vi "PLC.WriteValues.vi"(7 "Idx":i32, 8 "error in":errorcluster, 10 "Slot":i32, 11 "Data_in":T1={"Status"={"Idx"=0, "ConnRef"=0, "State"=enum."Off", "LiveBitTimer"=timestamp(0 s since 1904-01-01)}, "Sets"={"Enable"=FALSE, "IP"="", "Rack"=0, "Slot"=0, "LifeBitTimer_s"=0.0, "DataBlockAddr_PCStatus"=0, "DataBlockAddr_PLCStatus"=1, "DataBlockAddr_PLCNewData"=[], "DataBlockSize_PLCNewData"=[], "DataBlockAddr_PLCChangeOver"=[], "DataBlockSize_PLCChangeOver"=[], "DataBlockAddr_PCChangeOver"=[], "DataBlockAddr_PLCCheckStatus"=[], "DataBlockSize_PLCCheckStatus"=[], "DataBlockAddr_PCCheckStatus"=[], "System"=""}, "PCstatus"={"General"={"LifeBit"=FALSE, "DbRun"=FALSE}, "Stations"=[]}, "PLCstatus"={"General"={"LifeBit"=FALSE}, "Stations"=[]}}) -> (0 "error out":errorcluster, 3 "Data_out":T1={"Status"={"Idx"=0, "ConnRef"=0, "State"=enum."Off", "LiveBitTimer"=timestamp(0 s since 1904-01-01)}, "Sets"={"Enable"=FALSE, "IP"="", "Rack"=0, "Slot"=0, "LifeBitTimer_s"=0.0, "DataBlockAddr_PCStatus"=0, "DataBlockAddr_PLCStatus"=1, "DataBlockAddr_PLCNewData"=[], "DataBlockSize_PLCNewData"=[], "DataBlockAddr_PLCChangeOver"=[], "DataBlockSize_PLCChangeOver"=[], "DataBlockAddr_PCChangeOver"=[], "DataBlockAddr_PLCCheckStatus"=[], "DataBlockSize_PLCCheckStatus"=[], "DataBlockAddr_PCCheckStatus"=[], "System"=""}, "PCstatus"={"General"={"LifeBit"=FALSE, "DbRun"=FALSE}, "Stations"=[]}, "PLCstatus"={"General"={"LifeBit"=FALSE}, "Stations"=[]}})   [LabVIEW 2016]
doc: "Get test results (measurement values) from PLC and save to database\n\nWabco 2017 All right reserved\nAuthor: maciej.szupienko@wabco-auto.com"
uses:
  PLC.Data.ctl
  PLC.Data.Status.ctl
  PLC.State.ctl
  PLC.Data.Sets.ctl
  LowLevel/PLC.DataBlock.PCstatus.ctl
  LowLevel/PLC.DataBlock.PCstatus.General.ctl
  LowLevel/PLC.DataBlock.PCstatus.Station.ctl
  LowLevel/PLC.DataBlock.PLCstatus.ctl
  LowLevel/PLC.DataBlock.PLCstatus.General.ctl
  LowLevel/PLC.DataBlock.PLCstatus.Station.ctl
  LowLevel/PLC.DataBlock.PLCvalues.ctl
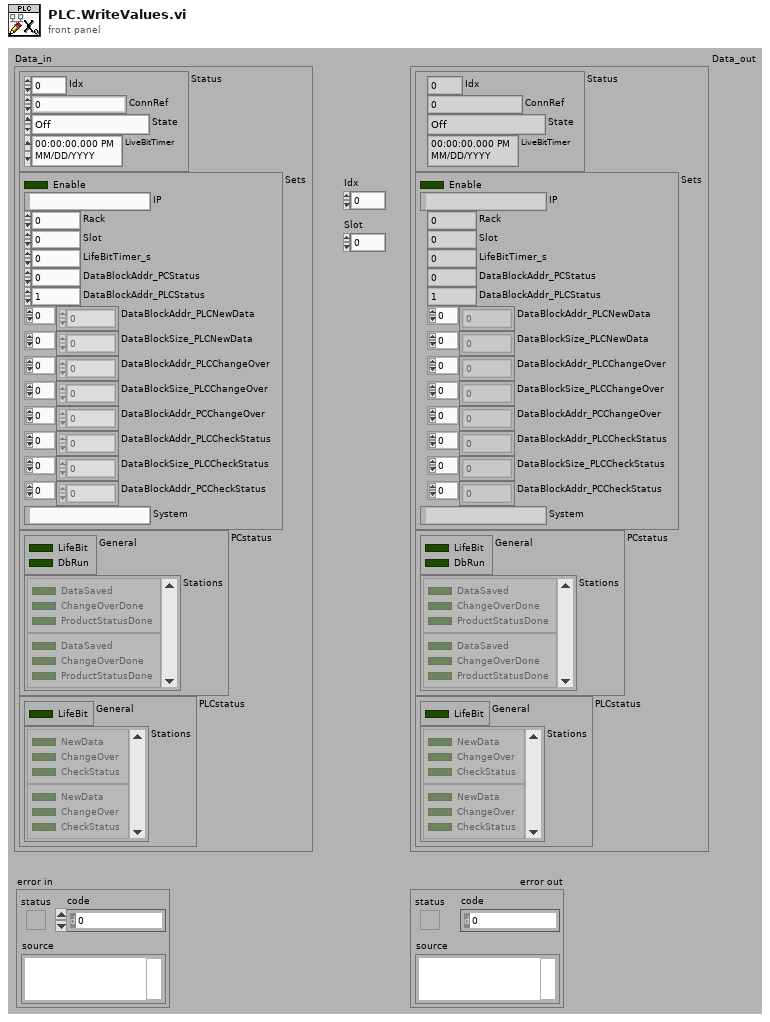
[diagram p1: front panel]
types:
  T1 = typedef "PLC.Data.ctl" = cluster{"Status":T2, "Sets":T4, "PCstatus":T5, "PLCstatus":T8}
  T2 = typedef "PLC.Data.Status.ctl" = cluster{"Idx":i32, "ConnRef":u64, "State":T3, "LiveBitTimer":timestamp}
  T3 = typedef "PLC.State.ctl" = enum32{"Off", "Error", "Idle", "Run"}
  T4 = typedef "PLC.Data.Sets.ctl" = cluster{"Enable":bool, "IP":string, "Rack":i32, "Slot":i32, "LifeBitTimer_s":dbl, "DataBlockAddr_PCStatus":i32, "DataBlockAddr_PLCStatus":i32, "DataBlockAddr_PLCNewData":i32[], "DataBlockSize_PLCNewData":i32[], "DataBlockAddr_PLCChangeOver":i32[], "DataBlockSize_PLCChangeOver":i32[], "DataBlockAddr_PCChangeOver":i32[], "DataBlockAddr_PLCCheckStatus":i32[], "DataBlockSize_PLCCheckStatus":i32[], "DataBlockAddr_PCCheckStatus":i32[], "System":string}
  T5 = typedef "PLC.DataBlock.PCstatus.ctl" = cluster{"General":T6, "Stations":T7[]}
  T6 = typedef "PLC.DataBlock.PCstatus.General.ctl" = cluster{"LifeBit":bool, "DbRun":bool}
  T7 = typedef "PLC.DataBlock.PCstatus.Station.ctl" = cluster{"DataSaved":bool, "ChangeOverDone":bool, "ProductStatusDone":bool}
  T8 = typedef "PLC.DataBlock.PLCstatus.ctl" = cluster{"General":T9, "Stations":T10[]}
  T9 = typedef "PLC.DataBlock.PLCstatus.General.ctl" = cluster{"LifeBit":bool}
  T10 = typedef "PLC.DataBlock.PLCstatus.Station.ctl" = cluster{"NewData":bool, "ChangeOver":bool, "CheckStatus":bool}
  T11 = typedef "PLC.DataBlock.PLCvalues.ctl" = cluster{"Status":u8, "Ref1":string, "Serial1":string, "Ref2":string, "Serial2":string, "Values":sgl[]}
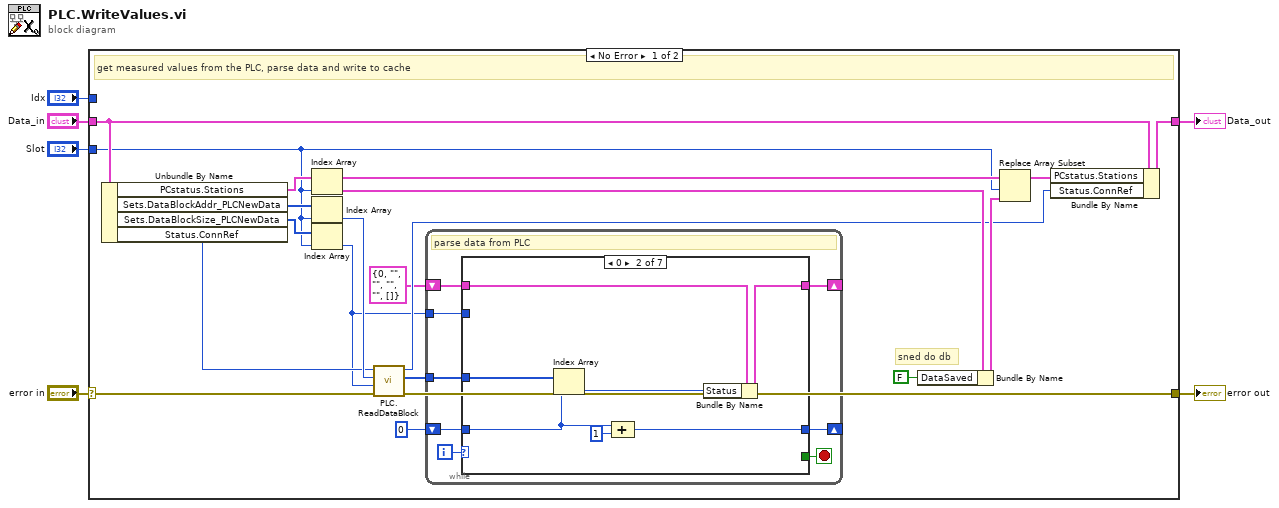
[diagram p0: block diagram]
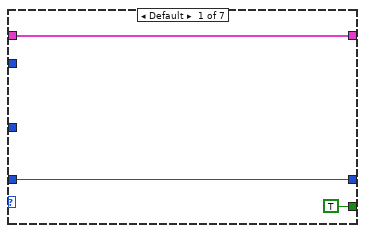
[diagram p2: hidden frame]
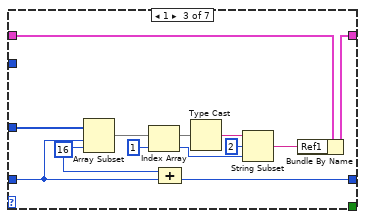
[diagram p3: hidden frame]
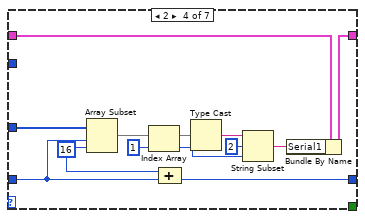
[diagram p4: hidden frame]
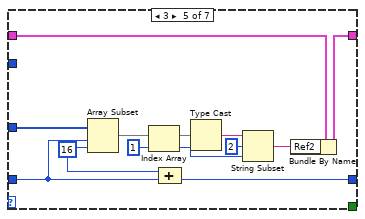
[diagram p5: hidden frame]
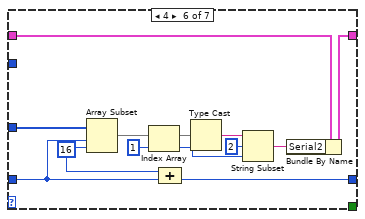
[diagram p6: hidden frame]
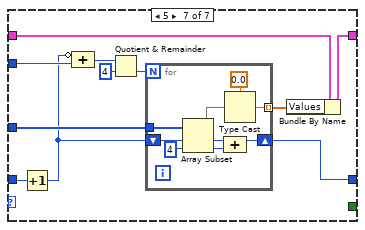
[diagram p7: hidden frame]
diagram:
  n1 = case shown="No Error" "error in" {
    selector: "error in" -> [w24 w111]
    tunnel: [w7 w111] -> w3
    tunnel: "Data_in" -> [w21 w110]
    tunnel: [w25 w110] -> w5
    tunnel: "Idx" -> [_ _]
    tunnel: "Slot" -> [w9 _]
    frame No Error {
      # "sned do db"
      # "get measured values from the PLC, parse data and write to cache"
      n2 = Unbundle By Name(w21) -> ("PCstatus.Stations"=w11:T7[], "Sets.DataBlockAddr_PLCNewData"=w23:i32[], "Sets.DataBlockSize_PLCNewData"=w10:i32[], "Status.ConnRef"=w20:u64)
      n3 = Index Array(array=w11, index=w9) -> (element=w18:T7)
      n4 = Index Array(array=w23, index=w9) -> (element=w22:i32)
      n5 = Index Array(array=w10, index=w9) -> (element=w12:i32)
      n6 = call "PLC.ReadDataBlock.vi"("error in (no error)"=w24, "Amount (1)"=w12, "Block"=w22, "Ref"=w20) -> ("error out"=w7:errorcluster, "data out"=w15:u8[], "ref out"=w16:u64)  [unwired: 5 in]
      n7 = while {
        tunnel: w15 -> [w28]
        shift-right: [w31] -> _
        shift-left: 0 -> [w32]
        shift-right: [w30] -> _
        shift-left: T11 {"Status"=0, "Ref1"="", "Serial1"="", "Ref2"="", "Serial2"="", "Values"=[]} ("element") -> [w29]
        tunnel: w12 -> [w27]
        i -> [w33]
        stop <- w26 stop-if-true
        # "parse data from PLC"
        n8 = case shown="0" w33 {
          tunnel: w32 -> [w35 w40 w46 w58 w70 w82 w93]
          tunnel: [w35 w41 w45 w57 w69 w81 w96] -> w31
          tunnel: [w36 w39 w55 w67 w79 w91 w101] -> w30
          tunnel: w29 -> [w36 w38 w54 w66 w78 w90 w102]
          tunnel: w28 -> [_ w43 w49 w61 w73 w85 w97]
          tunnel: w27 -> [_ _ _ _ _ _ w95]
          tunnel: [TRUE _ _ _ _ _ _] -> w26
          frame Default {
          }
          frame 0 {
            n9 = Index Array(array=w43, index=w40) -> (element=w42:u8)
            n10 = Compound Arithmetic op=ADD(w40, 1 ("value")) -> (w41:i32)
            n11 = Bundle By Name(cluster=w38, "Status"=w42) -> (w39:T11)
          }
          frame 1 {
            w47 = 16 ("length")
            n12 = Array Subset(array=w49, index=w46, length=w47) -> (w51:u8[])
            n13 = Index Array(array=w51, index=1) -> (element=w44:u8)
            n14 = Compound Arithmetic op=ADD(w47, w46) -> (w45:i32)
            n15 = Type Cast(x=w51) -> (*(type *) &x=w50:string)  [unwired: 1 in]
            n16 = String Subset(string=w50, offset (0)=2, length (rest)=w44) -> (substring=w48:string)
            n17 = Bundle By Name(cluster=w54, "Ref1"=w48) -> (w55:T11)
          }
          frame 2 {
            w59 = 16 ("length")
            n18 = Array Subset(array=w61, index=w58, length=w59) -> (w63:u8[])
            n19 = Index Array(array=w63, index=1) -> (element=w56:u8)
            n20 = Compound Arithmetic op=ADD(w59, w58) -> (w57:i32)
            n21 = Type Cast(x=w63) -> (*(type *) &x=w62:string)  [unwired: 1 in]
            n22 = String Subset(string=w62, offset (0)=2, length (rest)=w56) -> (substring=w60:string)
            n23 = Bundle By Name(cluster=w66, "Serial1"=w60) -> (w67:T11)
          }
          frame 3 {
            w71 = 16 ("length")
            n24 = Array Subset(array=w73, index=w70, length=w71) -> (w75:u8[])
            n25 = Index Array(array=w75, index=1) -> (element=w68:u8)
            n26 = Compound Arithmetic op=ADD(w71, w70) -> (w69:i32)
            n27 = Type Cast(x=w75) -> (*(type *) &x=w74:string)  [unwired: 1 in]
            n28 = String Subset(string=w74, offset (0)=2, length (rest)=w68) -> (substring=w72:string)
            n29 = Bundle By Name(cluster=w78, "Ref2"=w72) -> (w79:T11)
          }
          frame 4 {
            w83 = 16 ("length")
            n30 = Array Subset(array=w85, index=w82, length=w83) -> (w87:u8[])
            n31 = Index Array(array=w87, index=1) -> (element=w80:u8)
            n32 = Compound Arithmetic op=ADD(w83, w82) -> (w81:i32)
            n33 = Type Cast(x=w87) -> (*(type *) &x=w86:string)  [unwired: 1 in]
            n34 = String Subset(string=w86, offset (0)=2, length (rest)=w80) -> (substring=w84:string)
            n35 = Bundle By Name(cluster=w90, "Serial2"=w84) -> (w91:T11)
          }
          frame 5 {
            n36 = Increment(x=w93) -> (x+1=w92:i32)
            n37 = Compound Arithmetic op=ADD(invert w92, w95) -> (w100:i32)
            n38 = Quotient & Remainder(x=w100, y=4) -> (floor(x/y)=w94:i32)  [unwired: 1 out]
            n39 = for {
              N: w94 -> [_]
              shift-right: [w107] -> w96
              shift-left: w92 -> [w108]
              tunnel: w97 -> [w109]
              tunnel: [w104] -> w98 mode=indexing
              w106 = 4 ("length")
              n40 = Array Subset(array=w109, index=w108, length=w106) -> (w105:u8[])
              n41 = Compound Arithmetic op=ADD(w108, w106) -> (w107:i32)
              n42 = Type Cast(type=sgl 0.0 ("index"), x=w105) -> (*(type *) &x=w104:sgl)
            }
            n43 = Bundle By Name(cluster=w102, "Values"=w98) -> (w101:T11)
          }
        }
      }
      n44 = Bundle By Name(cluster=w18, "DataSaved"=FALSE) -> (w17:T7)
      n45 = Replace Array Subset(array=w11, new element=w17, index=w9) -> (w19:T7[])
      n46 = Bundle By Name(cluster=w21, "PCstatus.Stations"=w19, "Status.ConnRef"=w16) -> (w25:T1)
    }
    frame Error {
    }
  }
  "error out" <- w3
  "Data_out" <- w5
